vi "Write file.vi"(8 "error in (no error)":errorcluster, 9 "Logging Path":path, 10 "Color Parameters":T1, 11 "Metadata":string[][](array[string])) -> (0 "error out":errorcluster, 3 "file path out":path)   [LabVIEW 2013, in "AvaSpec Logging.lvlib"]
uses:
  AvaSpec Logging.lvlib
  Acquisition/AvaSpec Color Parameters.ctl
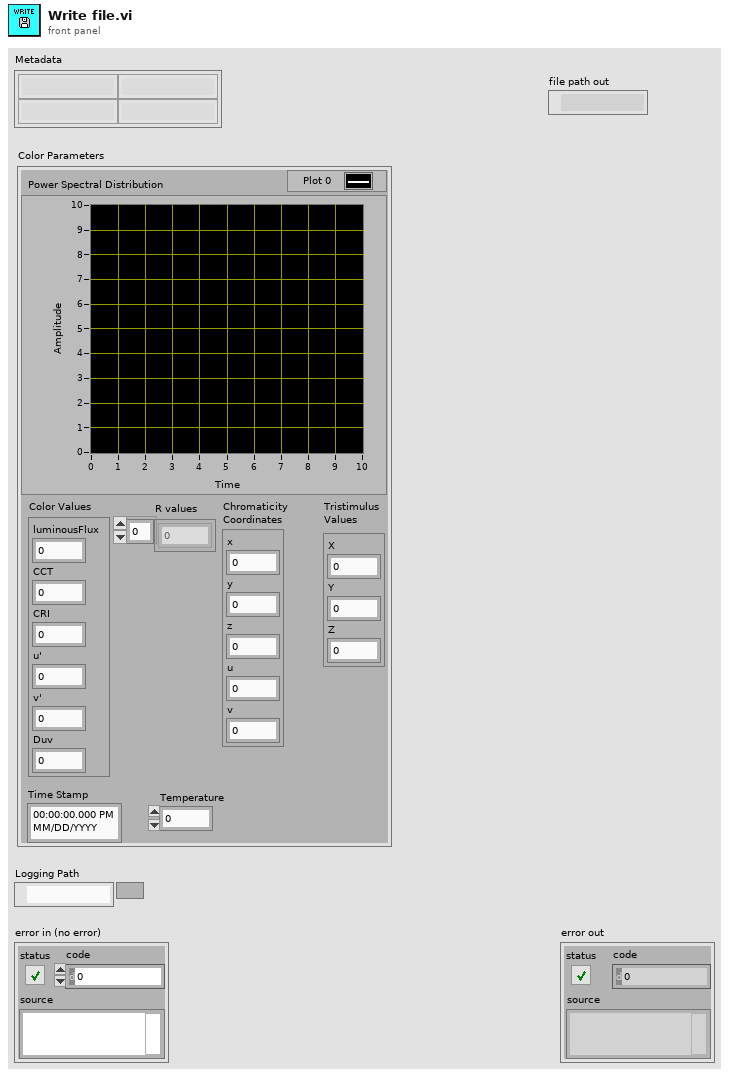
[diagram p1: front panel]
types:
  T1 = typedef "AvaSpec Color Parameters.ctl" = cluster{"Power Spectral Distribution":cluster{"X":dbl, "Y":dbl}[], "Color Values":cluster{"luminousFlux":dbl, "CCT":dbl, "CRI":dbl, "u'":dbl, "v'":dbl, "Duv":dbl}, "R values":dbl[], "Chromaticity \nCoordinates":cluster{"x":dbl, "y":dbl, "z":dbl, "u":dbl, "v":dbl}, "Tristimulus \nValues":cluster{"X":dbl, "Y":dbl, "Z":dbl}, "Time Stamp":timestamp, "Temperature":dbl}
  T2 = enum16{"open", "open or create", "create or replace", "create", "open (read-only)"}
  T3 = cluster{"luminousFlux":dbl, "CCT":dbl, "CRI":dbl, "u'":dbl, "v'":dbl, "Duv":dbl}
  T4 = cluster{"x":dbl, "y":dbl, "z":dbl, "u":dbl, "v":dbl}
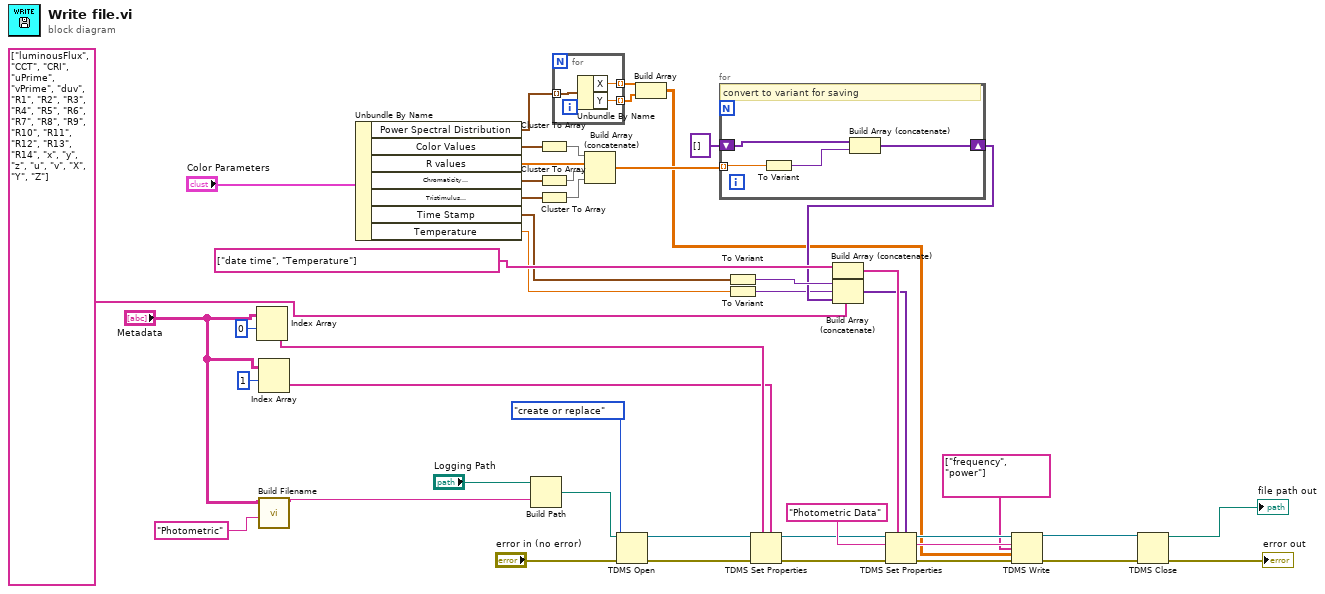
[diagram p0: block diagram]
diagram:
  n1 = Index Array(array="Metadata", index (row)=0) -> (element=w32:string[])  [unwired: 1 in]
  n2 = Index Array(array="Metadata", index (row)=1) -> (element=w31:string[])  [unwired: 1 in]
  n3 = call "Build Filename.vi"("Measurment Type"="Photometric", "Metadata In"="Metadata") -> ("String"=w3:string)  [unwired: 9 in]
  n4 = Unbundle By Name("Color Parameters") -> ("Power Spectral Distribution"=w11:cluster{"X":dbl, "Y":dbl}[], "Color Values"=w16:T3, "R values"=w14:dbl[], "Chromaticity \nCoordinates"=w20:T4, "Tristimulus \nValues"=w19:cluster{"X":dbl, "Y":dbl, "Z":dbl}, "Time Stamp"=w6:timestamp, "Temperature"=w5:dbl)
  n5 = Build Path(base path="Logging Path", name or relative path=w3) -> (appended path=w22:path)
  n6 = Cluster To Array(cluster=w16) -> (array=w15:dbl[])
  n7 = Cluster To Array(cluster=w20) -> (array=w18:dbl[])
  n8 = Cluster To Array(cluster=w19) -> (array=w17:dbl[])
  n9 = for {
    tunnel: w11 -> [w50] mode=indexing
    tunnel: [w49] -> w9 mode=indexing
    tunnel: [w48] -> w8 mode=indexing
    n10 = Unbundle By Name(w50) -> ("X"=w49:dbl, "Y"=w48:dbl)
  }
  n11 = Build Array (concatenate)(w15, w14, w18, w17) -> (w13:dbl[])
  n12 = TDMS Open(8:"error in (no error)", 10:T2."create or replace" ("operation (0:open)"), 11:w22) -> (0:w35:errorcluster, 3:w36:refnum<k34>)  [unwired: 4 in]
  n13 = Build Array(w9, w8) -> (w7:dbl[][])
  n14 = for {
    shift-right: [w54] -> w28
    shift-left: variant[] [] -> [w52]
    tunnel: w13 -> [w51] mode=indexing
    # "convert to variant for saving"
    n15 = To Variant(anything=w51) -> (Variant=w53:variant)
    n16 = Build Array (concatenate)(w52, w53) -> (w54:variant[])
  }
  n17 = To Variant(anything=w6) -> (Variant=w29:variant)
  n18 = To Variant(anything=w5) -> (Variant=w4:variant)
  n19 = TDMS Set Properties(5:w31, 7:w32, 8:w35, 11:w36) -> (0:w33:errorcluster, 3:w34:refnum<k34>)  [unwired: 2 in, 2 out]
  n20 = Build Array (concatenate)(string[] ["date time", "Temperature"] ("element"), string[] ["luminousFlux", "CCT", "CRI", "uPrime", "vPrime", "duv", "R1", "R2", "R3", "R4", "R5", "R6", "R7", "R8", "R9", "R10", "R11", "R12", "R13", "R14", "x", "y", "z", "u", "v", "X", "Y", "Z"]) -> (w42:string[])
  n21 = Build Array (concatenate)(w29, w4, w28) -> (w30:variant[])
  n22 = TDMS Set Properties(5:w30, 7:w42, 8:w33, 10:"Photometric Data" ("group name"), 11:w34) -> (0:w46:errorcluster, 2:w37:string, 3:w47:refnum<k34>)  [unwired: 1 in, 1 out]
  n23 = TDMS Write(0:w47, 5:w37, 7:string[] ["frequency", "power"] ("channel name(s) in (Untitled)"), 9:w7, 11:w46) -> (4:w45:refnum<k34>, 15:w44:errorcluster)  [unwired: 1 in, 2 out]
  n24 = TDMS Close(8:w44, 11:w45) -> (0:→"error out":errorcluster, 3:→"file path out":path)
